vi "ErrorAsk.vi"(8 "error in (no error)":errorcluster, 11 "VISA Refnum in":refnum<visa-resource-name>) -> (0 "error out":errorcluster, 3 "VISA Refnum out":refnum<visa-resource-name>)   [LabVIEW 2013]
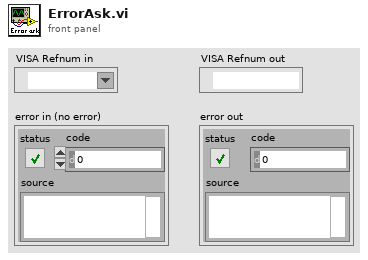
[diagram p1: front panel]
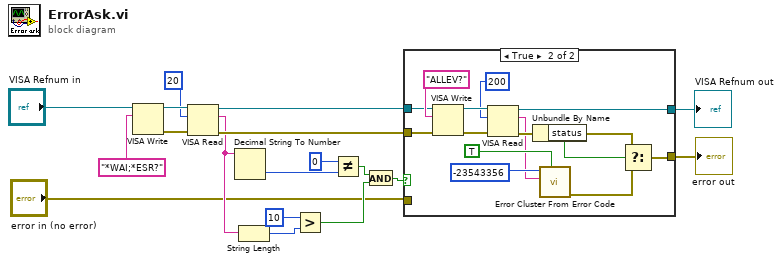
[diagram p0: block diagram]
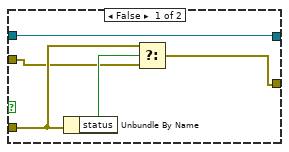
[diagram p2: hidden frame]
diagram:
  n1 = VISA Write(VISA resource name="VISA Refnum in", write buffer="*WAI;*ESR?") -> (VISA resource name out=w13:refnum<visa-resource-name>, error out=w12:errorcluster)  [unwired: 1 in, 1 out]
  n2 = VISA Read(VISA resource name=w13, byte count=u32 20, error in (no error)=w12) -> (VISA resource name out=w15:refnum<visa-resource-name>, read buffer=w8:string, error out=w16:errorcluster)  [unwired: 1 out]
  n3 = Decimal String To Number(string=w8) -> (number=w10:i32)  [unwired: 2 in, 1 out]
  n4 = String Length(string=w8) -> (length=w7:i32)
  n5 = Greater?(x=10, y=w7) -> (0:w3:bool)
  n6 = Not Equal?(x=0, y=w10) -> (x != y?=w4:bool)
  n7 = And(x=w4, y=w3) -> (x .and. y?=w5:bool)
  n8 = case shown="True" w5 {
    tunnel: w15 -> [w19 w33]
    tunnel: w16 -> [w21 w32]
    tunnel: "error in (no error)" -> [w22 _]
    tunnel: [w20 w25] -> w18
    tunnel: [w19 w24] -> w17
    frame False {
      n9 = Unbundle By Name(w22) -> ("status"=w23:bool)
      n10 = Select(t=w22, s=w23, f=w21) -> (s? t:f=w20:errorcluster)
    }
    frame True {
      n11 = VISA Write(VISA resource name=w33, write buffer="ALLEV?", error in (no error)=w32) -> (VISA resource name out=w36:refnum<visa-resource-name>, error out=w35:errorcluster)  [unwired: 1 out]
      n12 = VISA Read(VISA resource name=w36, byte count=u32 200, error in (no error)=w35) -> (VISA resource name out=w24:refnum<visa-resource-name>, read buffer=w26:string, error out=w28:errorcluster)  [unwired: 1 out]
      n13 = Unbundle By Name(w28) -> ("status"=w27:bool)
      n14 = call <vilib>:"Error Cluster From Error Code.vi"("show call chain? (False)"=TRUE, "error message (\"\")"=w26, "error code (0)"=-23543356) -> ("error out"=w31:errorcluster)  [unwired: 6 in]
      n15 = Select(t=w28, s=w27, f=w31) -> (s? t:f=w25:errorcluster)
    }
  }
  "error out" <- w18
  "VISA Refnum out" <- w17
